vi "Setup Switch Device.vi"(10 "Test Class in":refnum<class "Test Class.lvclass">, 11 "Instrument in":refnum<class "Instrument.lvclass">) -> (0 "error out":errorcluster)   [LabVIEW 2015, in "Instrument Setup.lvclass"]
uses:
  Instrument Setup.lvclass
  Classes/Instruments/Instrument/Class/Instrument.lvclass
  Test Class/Test Class.lvclass
  Classes/Instruments/Relay Control/Switch Executive/Switch Executive.lvclass
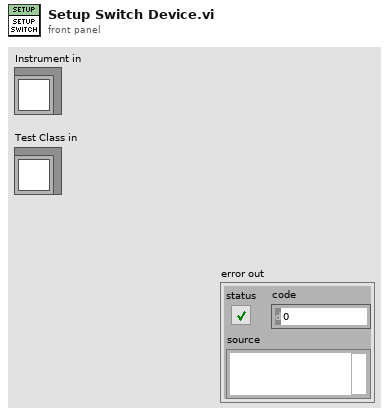
[diagram p1: front panel]
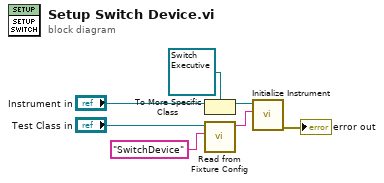
[diagram p0: block diagram]
diagram:
  n1 = To More Specific Class(target class=refnum<class "Switch Executive.lvclass"> refnum ("Switch Executive.lvlib:Switch Executive.lvclass"), reference="Instrument in") -> (specific class reference=w6:refnum<class "Switch Executive.lvclass">)  [unwired: 1 in, 1 out]
  n2 = call-dynamic "Read from Fixture Config.vi"("Key"="SwitchDevice" ("Name"), "Test Class in"="Test Class in") -> ("Instrument Info"=w1:string)  [unwired: 8 in, 1 out]
  n3 = call-dynamic "Initialize Instrument.vi"("Instrument Address"=w1, "Switch Executive in"=w6) -> ("error out"=→"error out":errorcluster)  [unwired: 8 in, 1 out]
